vi "Read Name - Returns Same Value.vi"() -> ()   [LabVIEW 2017, in "Cobertura.Tests.lvlib" / "Package.lvlib"]
uses:
  Package.lvlib
  Cobertura/Package/Package.lvclass/Package.ctl
  Cobertura/Package/Read Name.vi
  <vilib>/PNR/Transparent Assertions/Transparent Assertions/Transparent Assertions.lvlib
  Cobertura/Package/Package.lvclass
panel:
  out "error out":errorcluster
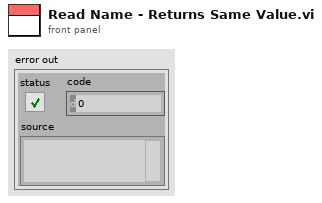
[diagram p1: front panel]
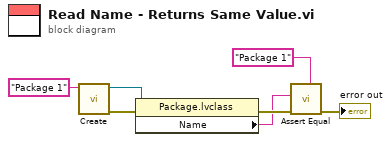
[diagram p0: block diagram]
diagram:
  n1 = call "Create.vi"("Name"="Package 1") -> ("error out"=w2:errorcluster, "Package"=w3:refnum<class "Package.lvclass">)  [unwired: 9 in]
  n2 = property class="Package.lvclass"(reference=w3, error in=w2) -> (error out=w7:errorcluster, "Name"=w5:string)  [unwired: 1 out]
  n3 = call <vilib>:"Assert Equal.vi"("Expected"="Package 1" ("Name"), "error in (no error)"=w7, "Actual"=w5) -> ("error out"=→"error out":errorcluster)  [unwired: 8 in]
